vi "save_log.vi"(8 "error in":errorcluster, 11 "ExperimentVariables in":refnum<class "ExperimentVariables.lvclass">) -> (0 "error out":errorcluster, 3 "ExperimentVariables out":refnum<class "ExperimentVariables.lvclass">)   [LabVIEW 2013]
uses:
  ExperimentVariables/ExperimentVariables.lvclass
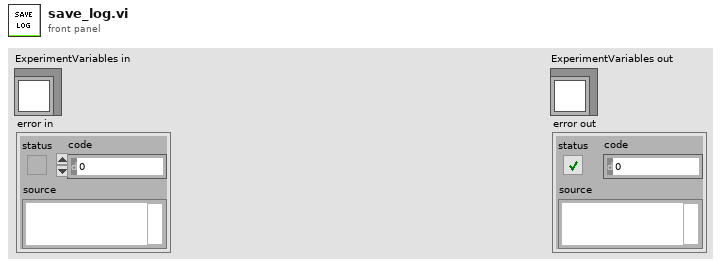
[diagram p1: front panel]
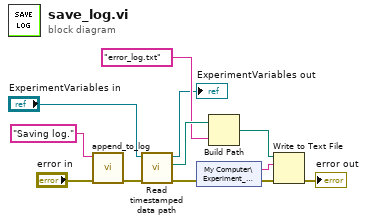
[diagram p0: block diagram]
diagram:
  n1 = call "append_to_log.vi"("error in"="error in", "string"="Saving log.") -> ("error out"=w11:errorcluster)  [unwired: 9 in]
  n2 = call-dynamic "Read timestamped data path.vi"("error in (no error)"=w11, "ExperimentVariables in"="ExperimentVariables in") -> ("error out"=w2:errorcluster, "Specific Data Files Path"=w10:path, "ExperimentVariables out"=→"ExperimentVariables out":refnum<class "ExperimentVariables.lvclass">)  [unwired: 7 in]
  n3 = shared-variable "My Computer\\Experiment_network_vars.lvlib\\Log"(error in=w2) -> (w3:string, error out=w1:errorcluster)
  n4 = Build Path(base path=w10, name or relative path="error_log.txt") -> (appended path=w9:path)
  n5 = Write to Text File(file (use dialog)=w9, text=w3, error in=w1) -> (error out=→"error out":errorcluster)  [unwired: 1 in, 2 out]
